vi "Yscale Set.vi"(8 "Log scale":dbl, 11 "Ref. Level":dbl) -> (0 "Y min":dbl, 3 "Y max":dbl)   [LabVIEW 2017]
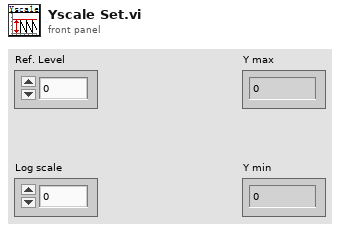
[diagram p1: front panel]
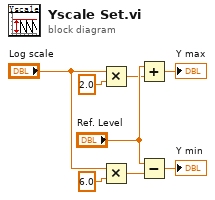
[diagram p0: block diagram]
diagram:
  n1 = Multiply(x="Log scale", y=2.0) -> (x*y=w4:dbl)
  n2 = Multiply(x="Log scale", y=6.0) -> (x*y=w3:dbl)
  n3 = Add(x="Ref. Level", y=w4) -> (x+y=→"Y max":dbl)
  n4 = Subtract(x="Ref. Level", y=w3) -> (x-y=→"Y min":dbl)
